vi "callController.vi"(8 "Error In":errorcluster, 9 "Simulation Module":bool[](array[boolean]), 10 "Application Path Cluster":T1, 11 "Software Name":string) -> (0 "Error Out":errorcluster)   [LabVIEW 2018]
uses:
  controls/pathCluster.ctl
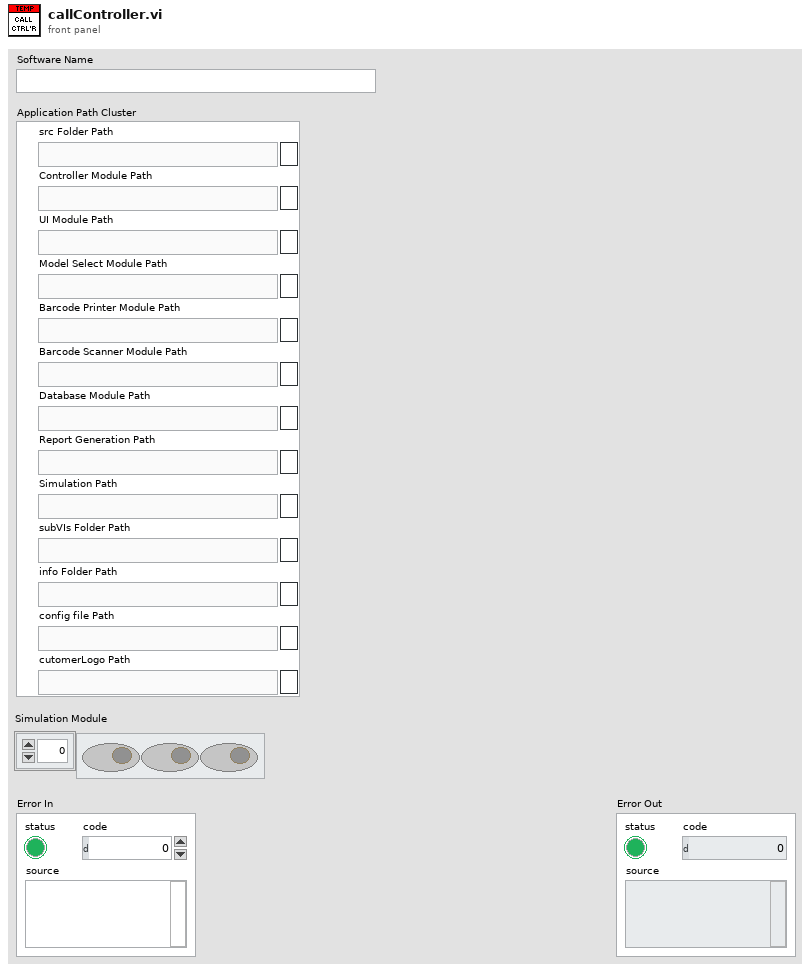
[diagram p1: front panel]
types:
  T1 = typedef "pathCluster.ctl" = cluster{"src Folder Path":path, "Controller Module Path":path, "UI Module Path":path, "Model Select Module Path":path, "Barcode Printer Module Path":path, "Barcode Scanner Module Path":path, "Database Module Path":path, "Report Generation Path":path, "Simulation Path":path, "subVIs Folder Path":path, "info Folder Path":path, "config file Path":path, "cutomerLogo Path":path}
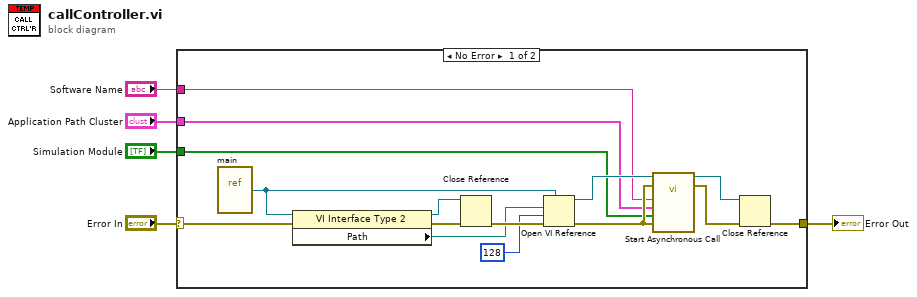
[diagram p0: block diagram]
diagram:
  n1 = case shown="No Error" "Error In" {
    selector: "Error In" -> [w20 w21]
    tunnel: [w8 w21] -> w4
    tunnel: "Software Name" -> [w11 _]
    tunnel: "Application Path Cluster" -> [w10 _]
    tunnel: "Simulation Module" -> [w6 _]
    frame No Error {
      n2 = vi-ref "main.vi"() -> (w13:refnum<vi>)
      n3 = property class="VI Interface Type 2"(reference=w13, error in=w20) -> (reference out=w18:refnum<vi>, error out=w19:errorcluster, "Path"=w16:path)
      n4 = Close Reference(reference=w18, error in (no error)=w19) -> (error out=w17:errorcluster)
      n5 = Open VI Reference(type specifier VI Refnum (for type only)=w13, vi path=w16, options=128, error in (no error)=w17) -> (vi reference=w14:refnum<vi>, error out=w12:errorcluster)  [unwired: 2 in]
      n6 = call-by-ref "Start Asynchronous Call"(reference=w14, error in=w12, "Error In"=w12, "Simulation Module"=w6, "Application Path Cluster"=w10, "Software Name"=w11) -> (reference out=w7:refnum<vi>, error out=w9:errorcluster)  [unwired: 7 in, 1 out]
      n7 = Close Reference(reference=w7, error in (no error)=w9) -> (error out=w8:errorcluster)
    }
    frame Error {
    }
  }
  "Error Out" <- w4
